vi "Constants.vi"() -> ()   [LabVIEW 2015, in "Fuel Injection Addon Shared.lvlib"]
doc: "Use this Global VI to access the GUIDs assigned to the page resources of the Custom Device."
uses:
  Fuel Injection Addon Shared.lvlib
panel:
  in  "Tab Control":enum32{"GUIDS", "Constants", "Properties"}(tab)=enum."Constants"
  in  "GUID.Stage Transition Setting":string="A8325CED-C5AD-4B11-973A-2D5825B320C2"
  in  "GUID.Pull In Transition Setting":string="1D0C00B4-381A-4E43-BECA-CB3D657DE24D"
  in  "GUID.Analysis Stage":string="198b8df0-5592-41d4-9531-c2ca5a908472"
  in  "GUID.FPGA Status":string="2c80e710-1dc5-4b49-b237-62e43c4c6177"
  in  "GUID.Fuel Injector Results Section":string="ab7bceb1-d71b-4408-9e3d-c8d84a29dda7"
  in  "GUID.Analysis Settings":string="033a2cfa-3dff-42aa-80d6-4d3b91cea342"
  in  "GUID.Delete Protected Channel":string="3bd3349d-9f32-45ed-b9ea-c744dd4a3418"
  in  "GUID.Fuel Injector Stage Section":string="8b8a8618-4ea0-4626-bd53-ac7957845392"
  in  "GUID.Global Settings":string="1a3b024c-1825-4e80-b0b5-31cd144714b0"
  in  "GUID.Fuel Injection Addon Disabled":string="ae00c97b-3405-44c3-be31-09e1af6209d0"
  in  "GUID.Fuel Injector Settings Section":string="e9154c6f-acef-45c9-a119-6d0b29a062da"
  in  "GUID.Fuel Injector Waveform Section":string="1aa0a4b2-2577-4b18-b578-5f1aebbfbe44"
  in  "GUID.Fuel Injector Shot Section":string="0405bd23-6654-460b-bd7a-21c2892e651a"
  in  "GUID.Fuel Injector Section":string="ee71788d-91e2-472e-ac53-a7227ffafe8e"
  in  "GUID.Fuel Injection Addon":string="ebb85750-2082-4125-b2c9-f3250be8ebcb"
  in  "StageSettings.DwellLevel":string="Dwell Level"
  in  "Constants.Injector.Stage.NumberFound":string="Found Stages"
  in  "GlobalSettings.InitialVoltageThreshold":string="Initial Voltage Threshold"
  in  "Constants.ExpectedTransitionsPerStage":u32=3
  in  "Constants.Injector.Settings.Current.Offset":string="Current Offset"
  in  "GlobalSettings.Current.Gain":string="Current Gain"
  in  "GlobalSettings.Volt.Gain":string="Voltage Gain"
  in  "Constants.GlobalSettings.Analysis Section":string="Analysis Settings"
  in  "Constants.Injector.Shot.Stage Section Name":string="Stage"
  in  "Constants.Injector.Event Time":string="Injection Event Time"
  in  "Constants.Injector.Settings.Volt.Offset":string="Voltage Offset"
  in  "Constants.Injector.Event Count":string="Injection Event Count"
  in  "Constants.Injector.Period":string="Injection Period"
  in  "GlobalSettings.InjectionDuration":string="Injection Duration"
  in  "GlobalSettings.Name":string="Global Settings"
  in  "GlobalSettings.EnableCapture":string="Enable Injection Capture"
  in  "Constants.Injector.Settings.Stream Wfms?":string="Stream waveform?"
  in  "Constants.Injector.Settings.Section Name":string="Settings"
  in  "Constants.Injector.Wfm.Current Wfm Channel Name":string="Current Waveform"
  in  "Constants.Injector.Wfm.Voltage Wfm Channel Name":string="Voltage Waveform"
  in  "Constants.Injector.Shot.Section Name":string="Shot"
  in  "Constants.Injector.Wfm.Section Name":string="Waveforms"
  in  "Constants.Injector.Shot.Duration":string="Shot Time"
  in  "Constants.Injector.Results.Section Name":string="Results"
  in  "Constants.Fuel Injector Add-on Name":string="Fuel Injection Add-on"
  in  "Constants.RTBitfileBasePath":string="c:\\ni-rt\\VeriStand\\Custom Devices\\Fuel Injection Addon"
  in  "ChannelGroup.FindStages":string="FindStages"
  in  "Properties.Injector.Waveforms":string="Injector.Waveforms"
  in  "Properties.Stage.Transition":string="Stage.Transition"
  in  "Properties.PullIn.Type":string="PullIn.Type"
  in  "Properties.Injector Timeout":string="Injector Timeout"
  in  "Properties.Channel.OriginalName":string="OriginalName"
  in  "Properties.Stages":string="Stages"
  in  "Properties.Mux.Register":string="FPGA Mux Register"
  in  "Properties.Timing.Register":string="FPGA Timing Register"
  in  "ChannelGroup.FPGAStatus":string="FPGAStatus"
  in  "Properties.FPGA.Register":string="FPGA Register"
  in  "ChannelGroup.Results":string="Results"
  in  "ChannelGroup.WaveformEnable":string="WaveformEnable"
  in  "ChannelGroup.DetectionSettings":string="PeakAndValleyDetection"
  in  "Properties.DMA.Name":string="InjectorDataDMA"
  in  "Properties.DependentFile.Bitfile":string="Bitfile"
  in  "Properties.Path.RTBitfilePath":string="RTBitfilePath"
  in  "Properties.U16.InjectorCount":string="InjectorCount"
  in  "Properties.Compiled.Settings":string="Settings"
  in  "Properties.String.DMAName":string="DMAName"
  in  "Properties.U32.SampleRate":string="SampleRate"
  in  "Properties.String.DeviceAddress":string="DeviceAddress"
  in  "Properties.Path.LocalBitfilePath":string="LocalBitfilePath"
  in  "Properties.MaxShots":string="Max Inj Shot Count"
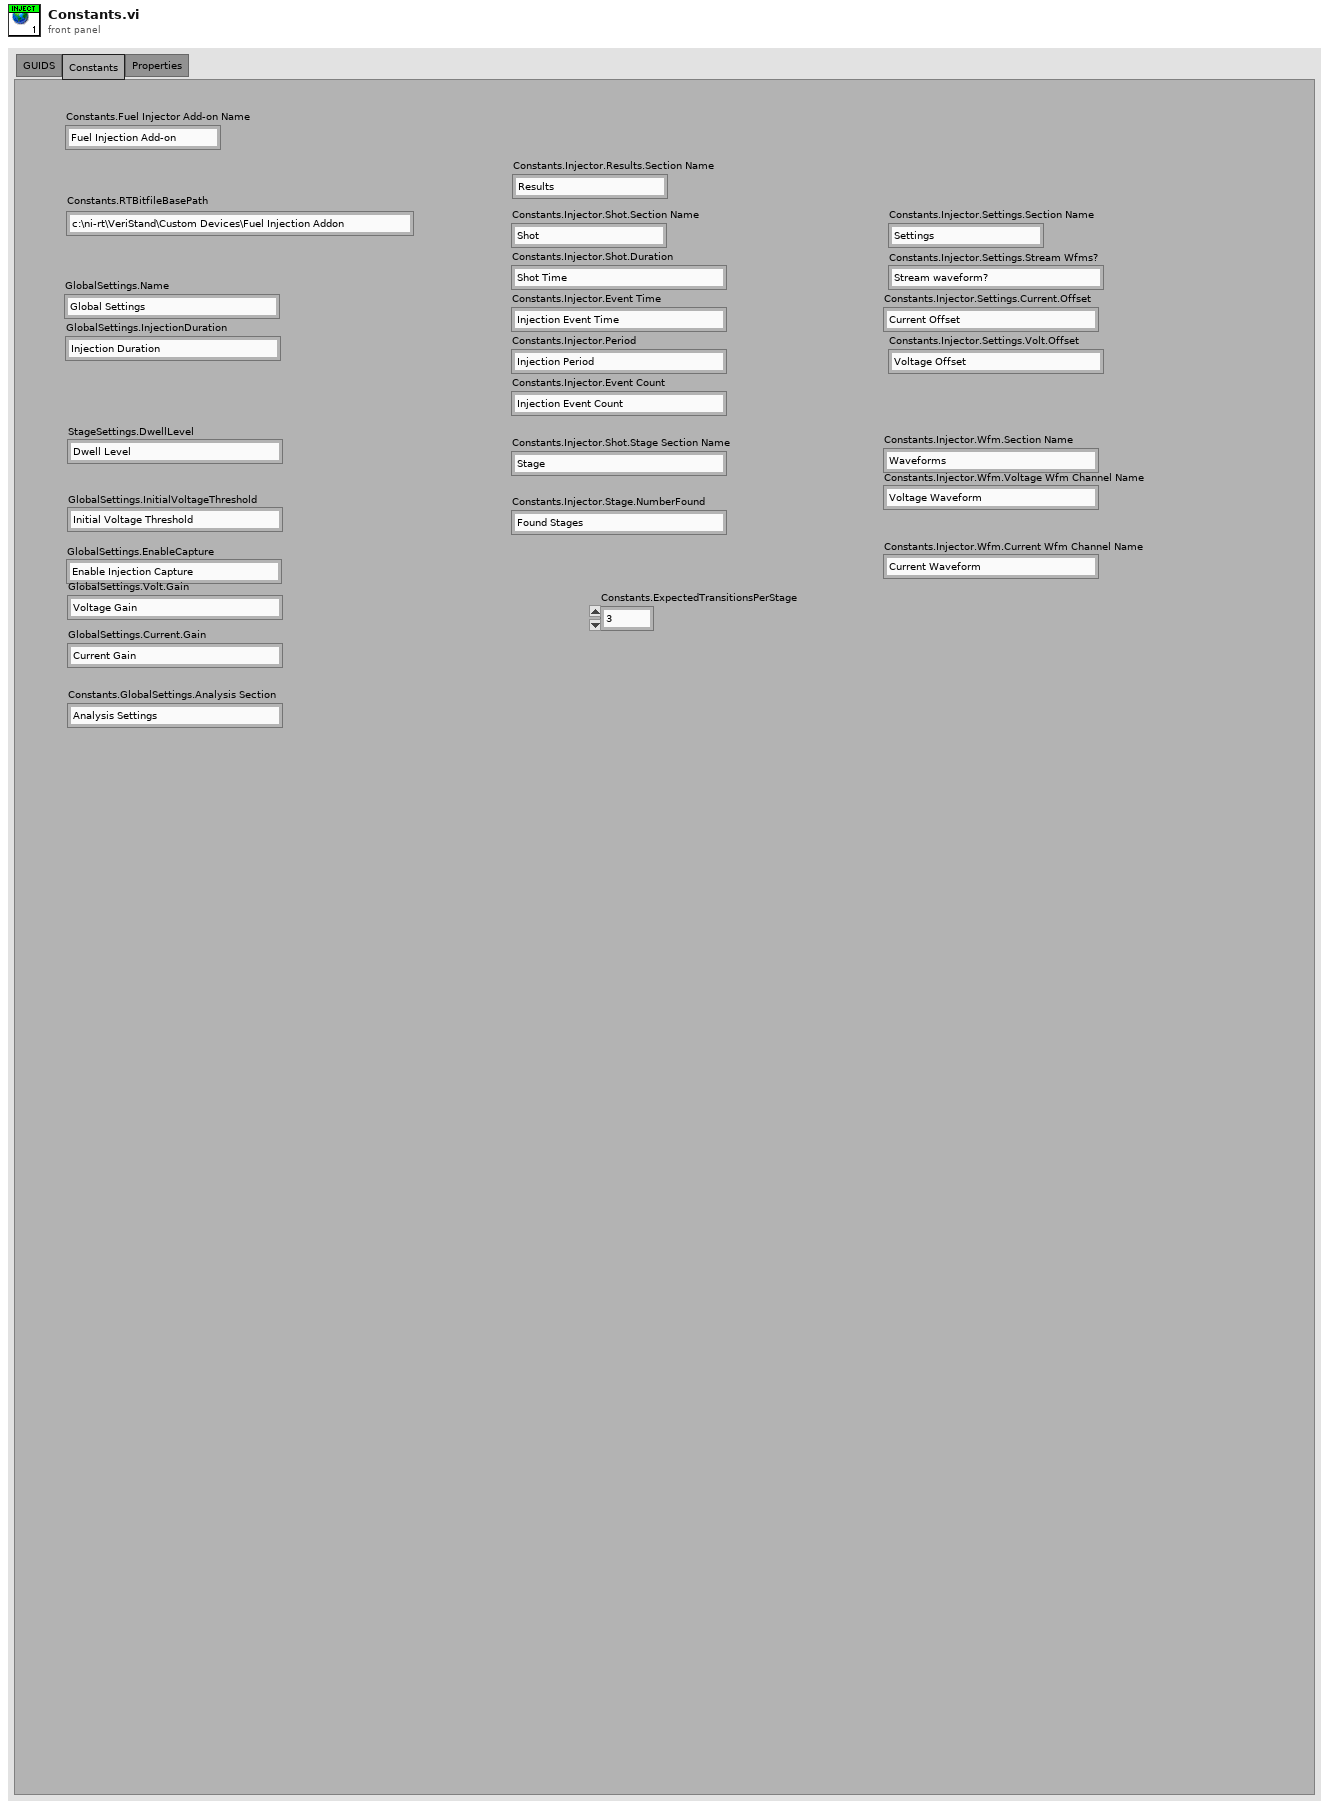
[diagram p1: front panel]
diagram:
